vi "EJERCICIO 4.vi"() -> ()   [LabVIEW 2012]
panel:
  in  "TOLERANCIA":string(combo)
  in  "3° FRANJA":string(combo)
  in  "2° FRANJA":string(combo)
  in  "1 ° FRANJA":string(combo)
  out "Color Box 4":u32(colorbox)
  out "Color Box 3":u32(colorbox)
  out "Color Box 2":u32(colorbox)
  out "Color Box":u32(colorbox)
  out "TOLERANCIA":string
  out "VALOR EDE LA RESISTENCIA":dbl
  in  "stop":bool
  # "INGRESE LOS COLORES"
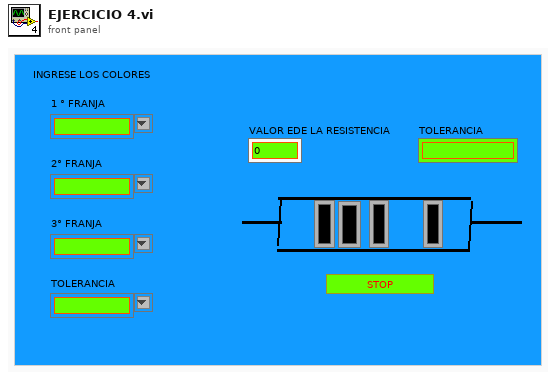
[diagram p1: front panel]
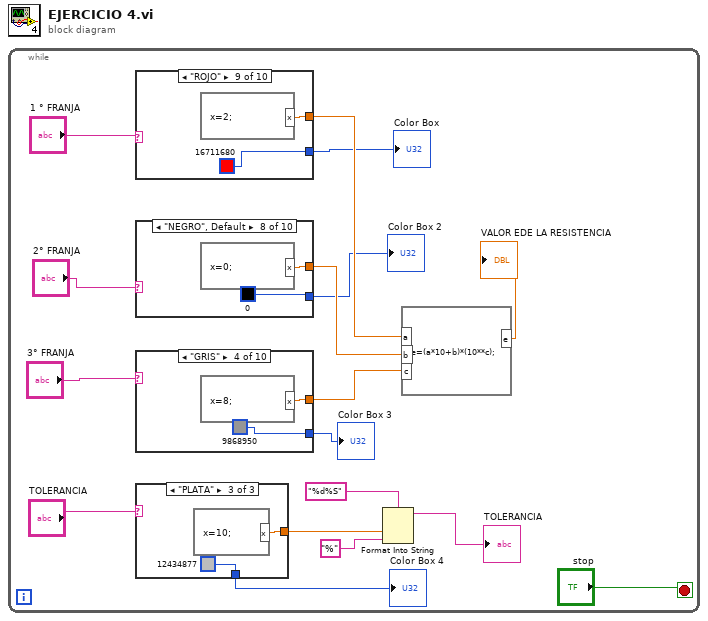
[diagram p0: block diagram]
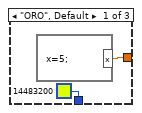
[diagram p2: hidden frame]
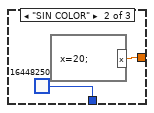
[diagram p3: hidden frame]
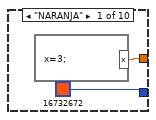
[diagram p4: hidden frame]
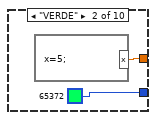
[diagram p5: hidden frame]
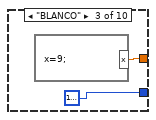
[diagram p6: hidden frame]
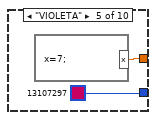
[diagram p7: hidden frame]
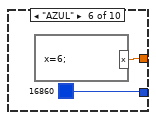
[diagram p8: hidden frame]
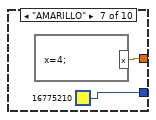
[diagram p9: hidden frame]
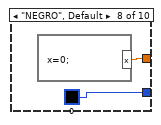
[diagram p10: hidden frame]
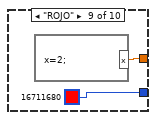
[diagram p11: hidden frame]
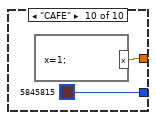
[diagram p12: hidden frame]
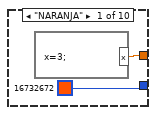
[diagram p13: hidden frame]
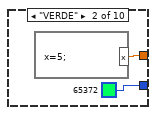
[diagram p14: hidden frame]
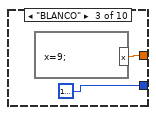
[diagram p15: hidden frame]
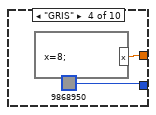
[diagram p16: hidden frame]
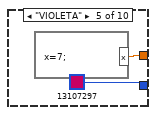
[diagram p17: hidden frame]
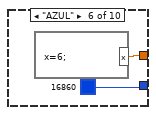
[diagram p18: hidden frame]
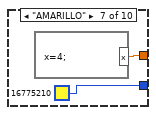
[diagram p19: hidden frame]
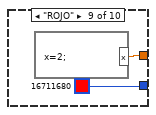
[diagram p20: hidden frame]
diagram:
  n1 = while {
    stop <- "stop" stop-if-true
    n2 = case shown="\"ROJO\"" "1 ° FRANJA" {
      tunnel: [w65 w67 w69 w71 w73 w75 w77 w79 w81 w83] -> w17
      tunnel: [u32 16732672 ("Color Box") u32 65372 ("Color Box") u32 16777238 ("Color Box") u32 9868950 ("Color Box") u32 13107297 ("Color Box") u32 16860 ("Color Box") u32 16775210 ("Color Box") u32 0 ("Color Box") u32 16711680 ("Color Box") u32 5845815 ("Color Box")] -> w9
      frame "NARANJA" {
        n3 = formula code="x=3;"() -> ("x"=w65:dbl)
      }
      frame "VERDE" {
        n4 = formula code="x=5;"() -> ("x"=w67:dbl)
      }
      frame "BLANCO" {
        n5 = formula code="x=9;"() -> ("x"=w69:dbl)
      }
      frame "GRIS" {
        n6 = formula code="x=8;"() -> ("x"=w71:dbl)
      }
      frame "VIOLETA" {
        n7 = formula code="x=7;"() -> ("x"=w73:dbl)
      }
      frame "AZUL" {
        n8 = formula code="x=6;"() -> ("x"=w75:dbl)
      }
      frame "AMARILLO" {
        n9 = formula code="x=4;"() -> ("x"=w77:dbl)
      }
      frame "NEGRO", Default {
        n10 = formula code="x=0;"() -> ("x"=w79:dbl)
      }
      frame "ROJO" {
        n11 = formula code="x=2;"() -> ("x"=w81:dbl)
      }
      frame "CAFE" {
        n12 = formula code="x=1;"() -> ("x"=w83:dbl)
      }
    }
    "Color Box" <- w9
    n13 = case shown="\"NEGRO\", Default" "2° FRANJA" {
      tunnel: [w45 w47 w49 w51 w53 w55 w57 w59 w61 w63] -> w16
      tunnel: [u32 16732672 ("Color Box") u32 65372 ("Color Box") u32 16777238 ("Color Box") u32 9868950 ("Color Box") u32 13107297 ("Color Box") u32 16860 ("Color Box") u32 16775210 ("Color Box") u32 0 ("Color Box") u32 16711680 ("Color Box") u32 5845815 ("Color Box")] -> w8
      frame "NARANJA" {
        n14 = formula code="x=3;"() -> ("x"=w45:dbl)
      }
      frame "VERDE" {
        n15 = formula code="x=5;"() -> ("x"=w47:dbl)
      }
      frame "BLANCO" {
        n16 = formula code="x=9;"() -> ("x"=w49:dbl)
      }
      frame "GRIS" {
        n17 = formula code="x=8;"() -> ("x"=w51:dbl)
      }
      frame "VIOLETA" {
        n18 = formula code="x=7;"() -> ("x"=w53:dbl)
      }
      frame "AZUL" {
        n19 = formula code="x=6;"() -> ("x"=w55:dbl)
      }
      frame "AMARILLO" {
        n20 = formula code="x=4;"() -> ("x"=w57:dbl)
      }
      frame "NEGRO", Default {
        n21 = formula code="x=0;"() -> ("x"=w59:dbl)
      }
      frame "ROJO" {
        n22 = formula code="x=2;"() -> ("x"=w61:dbl)
      }
      frame "CAFE" {
        n23 = formula code="x=1;"() -> ("x"=w63:dbl)
      }
    }
    "Color Box 2" <- w8
    n24 = case shown="\"GRIS\"" "3° FRANJA" {
      tunnel: [w25 w27 w29 w31 w33 w35 w37 w39 w41 w43] -> w15
      tunnel: [u32 16732672 ("Color Box") u32 65372 ("Color Box") u32 16777238 ("Color Box") u32 9868950 ("Color Box") u32 13107297 ("Color Box") u32 16860 ("Color Box") u32 16775210 ("Color Box") u32 0 ("Color Box") u32 16711680 ("Color Box") u32 5845815 ("Color Box")] -> w7
      frame "NARANJA" {
        n25 = formula code="x=3;"() -> ("x"=w25:dbl)
      }
      frame "VERDE" {
        n26 = formula code="x=5;"() -> ("x"=w27:dbl)
      }
      frame "BLANCO" {
        n27 = formula code="x=9;"() -> ("x"=w29:dbl)
      }
      frame "GRIS" {
        n28 = formula code="x=8;"() -> ("x"=w31:dbl)
      }
      frame "VIOLETA" {
        n29 = formula code="x=7;"() -> ("x"=w33:dbl)
      }
      frame "AZUL" {
        n30 = formula code="x=6;"() -> ("x"=w35:dbl)
      }
      frame "AMARILLO" {
        n31 = formula code="x=4;"() -> ("x"=w37:dbl)
      }
      frame "NEGRO", Default {
        n32 = formula code="x=0;"() -> ("x"=w39:dbl)
      }
      frame "ROJO" {
        n33 = formula code="x=2;"() -> ("x"=w41:dbl)
      }
      frame "CAFE" {
        n34 = formula code="x=1;"() -> ("x"=w43:dbl)
      }
    }
    "Color Box 3" <- w7
    n35 = case shown="\"PLATA\"" "TOLERANCIA" {
      tunnel: [w19 w21 w23] -> w12
      tunnel: [u32 14483200 ("Color Box") u32 16448250 ("Color Box") u32 12434877 ("Color Box")] -> w6
      frame "ORO", Default {
        n36 = formula code="x=5;"() -> ("x"=w19:dbl)
      }
      frame "SIN COLOR" {
        n37 = formula code="x=20;"() -> ("x"=w21:dbl)
      }
      frame "PLATA" {
        n38 = formula code="x=10;"() -> ("x"=w23:dbl)
      }
    }
    "Color Box 4" <- w6
    n39 = Format Into String "Format Into String"(format string="%d%S", w12, "%" ("format string")) -> (resulting string=→"TOLERANCIA":string)  [unwired: 2 in, 1 out]
    n40 = formula code="e=(a*10+b)*(10**c);"("a"=w17, "c"=w15, "b"=w16) -> ("e"=→"VALOR EDE LA RESISTENCIA":dbl)
  }
